vi "DeleteAcc.vi"(8 "error in (no error)":errorcluster, 11 "UserManagement in":refnum<class "UserManagement.lvclass">) -> (0 "error out":errorcluster, 3 "UserManagement out":refnum<class "UserManagement.lvclass">)   [LabVIEW 2019, in "UserManagement.lvlib" / "UserManagement.lvclass"]
uses:
  UserManagement.lvclass
  UserManagement.lvclass/UserManagement.ctl
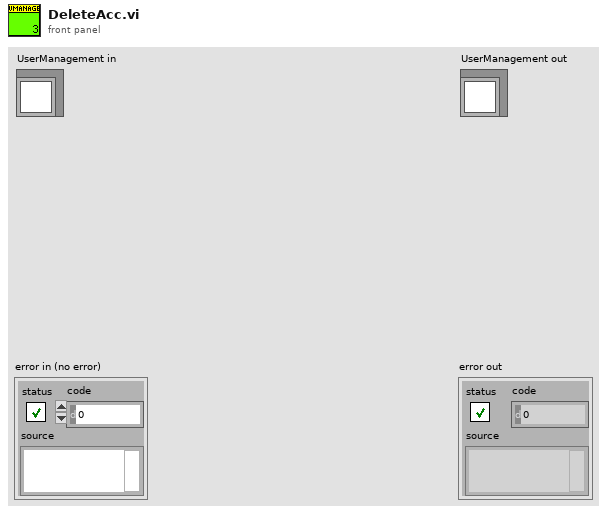
[diagram p1: front panel]
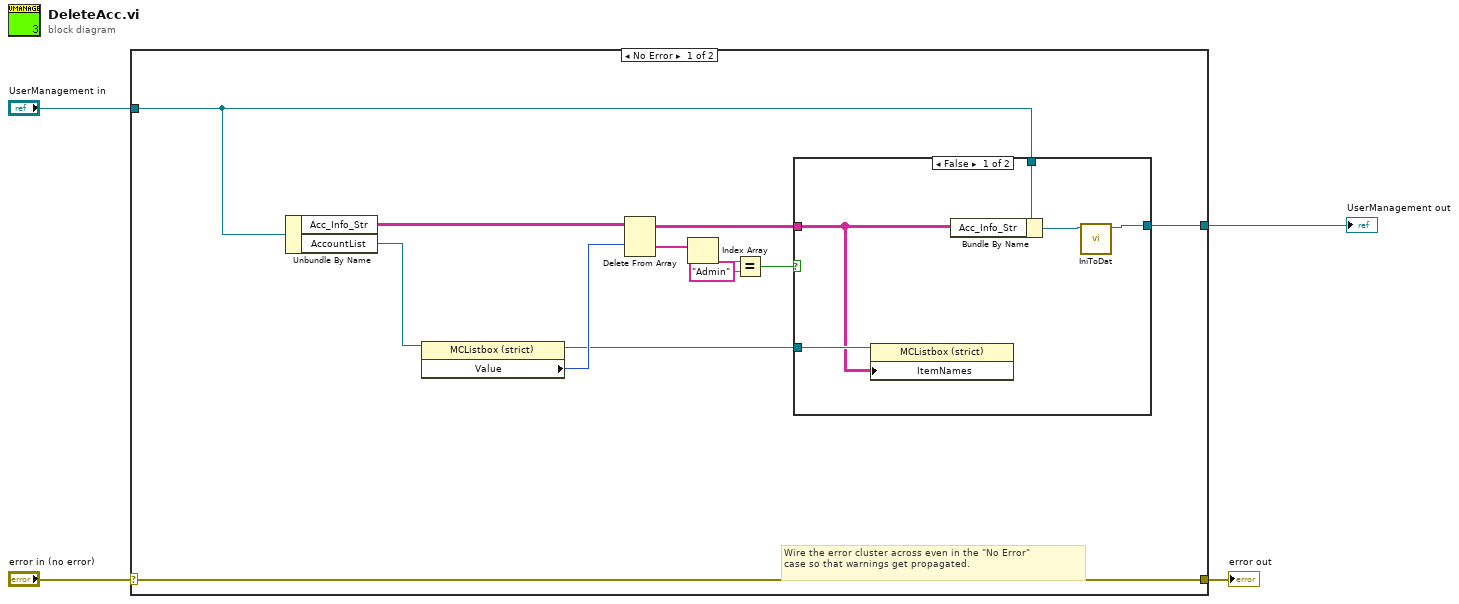
[diagram p0: block diagram]
diagram:
  n1 = case shown="No Error" "error in (no error)" {
    selector: "error in (no error)" -> [w16 w24]
    tunnel: [w16 w24] -> w3
    tunnel: [w9 w23] -> w1
    tunnel: "UserManagement in" -> [w10 w23]
    frame No Error {
      # "Wire the error cluster across even in the \"No Error\"\ncase so that warnings get propagated."
      n2 = Unbundle By Name(w10) -> ("Acc_Info_Str"=w14:string[][], "AccountList"=w15:refnum<vi>)
      n3 = property class="MCListbox (strict)"(reference=w15) -> (reference out=w12:refnum<vi>, "Value"=w13:i32)  [unwired: 1 in, 1 out]
      n4 = Delete From Array(array=w14, index (row)=w13) -> (deleted portion=w8:string[], array with subset deleted=w11:string[][])  [unwired: 2 in]
      n5 = Index Array(array=w8) -> (element=w7:string)  [unwired: 1 in]
      n6 = Equal?(x=w7, y="Admin") -> (x = y?=w5:bool)
      n7 = case shown="False" w5 {
        tunnel: w12 -> [w21 _]
        tunnel: w11 -> [w20 _]
        tunnel: w10 -> [w19 w22]
        tunnel: [w17 w22] -> w9
        frame False {
          n8 = property class="MCListbox (strict)"(reference=w21, "ItemNames"=w20) -> ()  [unwired: 1 in, 2 out]
          n9 = Bundle By Name(cluster=w19, "Acc_Info_Str"=w20) -> (w18:refnum<class "UserManagement.lvclass">)
          n10 = call-dynamic "IniToDat.vi"("UserManagement in"=w18) -> ("UserManagement out"=w17:refnum<class "UserManagement.lvclass">)  [unwired: 9 in, 1 out]
        }
        frame True {
        }
      }
    }
    frame Error {
    }
  }
  "error out" <- w3
  "UserManagement out" <- w1
